vi "Get Tolerance String (SubVI).vi"(10 "Tolerance Value":dbl) -> (2 "Tolerance String":string)   [LabVIEW 2011]
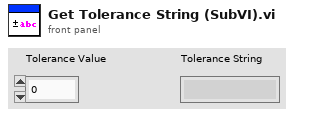
[diagram p1: front panel]
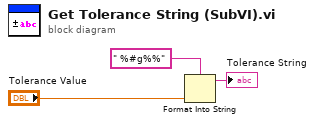
[diagram p0: block diagram]
diagram:
  n1 = Format Into String(format string=" %#g%%", "Tolerance Value") -> (resulting string=→"Tolerance String":string)  [unwired: 2 in, 1 out]
